vi "NDMotor_MoveForward.vi"(8 "error in":errorcluster, 10 "Steps":i32, 11 "VISA resource name":refnum<visa-resource-name>) -> (0 "error out":errorcluster, 1 "move time (ms)":i32, 2 "steps":i32, 3 "VISA resource name out":refnum<visa-resource-name>)   [LabVIEW 2024]
panel:
  out "read buffer":string
  out "concatenated string":string
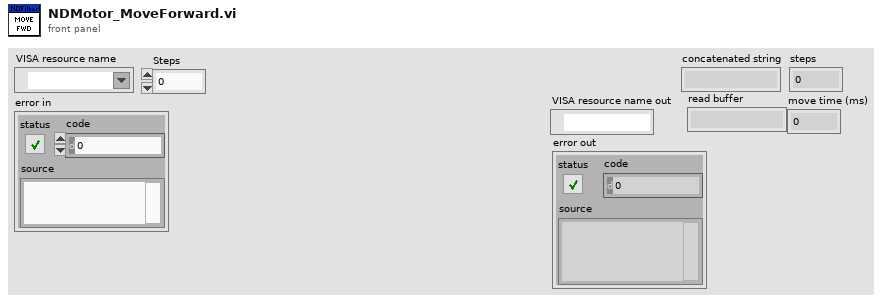
[diagram p1: front panel]
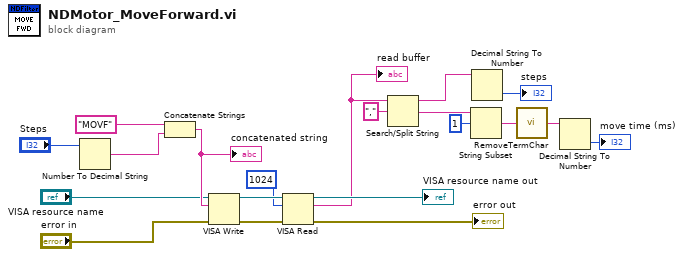
[diagram p0: block diagram]
diagram:
  n1 = Number To Decimal String(number="Steps") -> (decimal integer string=w17:string)  [unwired: 1 in]
  n2 = Concatenate Strings("MOVF", w17) -> (w19:string)
  "concatenated string" <- w19
  n3 = VISA Write(VISA resource name="VISA resource name", write buffer=w19, error in (no error)="error in") -> (VISA resource name out=w14:refnum<visa-resource-name>, error out=w13:errorcluster)  [unwired: 1 out]
  n4 = VISA Read(VISA resource name=w14, byte count=u32 1024, error in (no error)=w13) -> (VISA resource name out=→"VISA resource name out":refnum<visa-resource-name>, read buffer=w9:string, error out=→"error out":errorcluster)  [unwired: 1 out]
  "read buffer" <- w9
  n5 = Search/Split String(string=w9, search string/char (-)=",") -> (substring before match=w4:string, match + rest of string=w7:string)  [unwired: 1 in, 1 out]
  n6 = String Subset(string=w7, offset (0)=1) -> (substring=w5:string)  [unwired: 1 in]
  n7 = Decimal String To Number(string=w4) -> (number=→"steps":i32)  [unwired: 2 in, 1 out]
  n8 = call "RemoveTermChar.vi"("String"=w5) -> ("Chopped String"=w2:string)  [unwired: 4 in]
  n9 = Decimal String To Number(string=w2) -> (number=→"move time (ms)":i32)  [unwired: 2 in, 1 out]
